vi "Facade.vi"(0 "Data In":T6, 2 "Display State In":T2, 3 "Container State":T5) -> (6 "Data Out":T6, 7 "Display State Out":T2, 8 "Action":T1)   [LabVIEW 2017, in "UI_TimeSelector.xctl"]
uses:
  UI_TimeSelector.xctl
  Data.ctl
  <vilib>/_xctls/Container State.ctl
  State.ctl
  Typedefs/INTERNAL-DATA.ctl
  Interface/DEF-Mode.ctl
  <vilib>/_xctls/Action.ctl
  Typedefs/INTERNAL-REFs.ctl
  <vilib>/_xctls/XControlSupport.lvlib
panel:
  in  "Second":string(combo)
  in  "Year":string(combo)
  in  "Month":string(combo)
  in  "Day":string(combo)
  in  "Hour":string(combo)
  in  "Minute":string(combo)
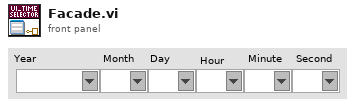
[diagram p1: front panel]
types:
  T1 = typedef "XControlSupport.lvlib/Action.ctl" = cluster{"Data Changed?":bool, "State Changed?":bool, "Action Name":string}
  T2 = typedef "UI_TimeSelector.xctl/State.ctl" = cluster{"data":T3, "mode":T4}
  T3 = typedef "UI_TimeSelector.xctl/INTERNAL-DATA.ctl" = cluster{"year":string, "month":string, "day":string, "hour":string, "minute":string, "second":string}
  T4 = typedef "UI_TimeSelector.xctl/DEF-Mode.ctl" = enum16{"YYYYMMDDHHMM", "YYYYMMDDHHMMSS", "YYYY", "YYYYMM", "YYYYMMDD", "HHMM", "HHMMSS"}
  T5 = typedef "XControlSupport.lvlib/Container State.ctl" = cluster{"Indicator?":bool, "Run Mode?":bool, " Refnum":refnum<vi>}
  T6 = typedef "UI_TimeSelector.xctl/Data.ctl" = timestamp
  T7 = typedef "UI_TimeSelector.xctl/INTERNAL-REFs.ctl" = cluster{"Year":refnum<vi>, "Month":refnum<vi>, "Day":refnum<vi>, "Hour":refnum<vi>, "Minute":refnum<vi>, "Second":refnum<vi>}
  T8 = cluster{"Year":string, "Month":string, "Day":string, "Hour":string, "Minute":string, "Second":string}
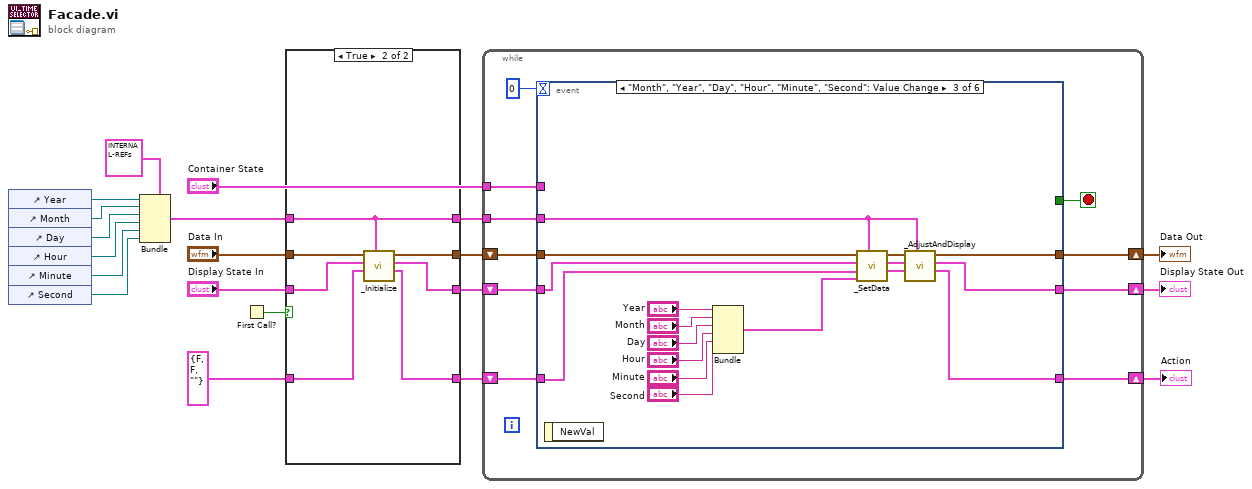
[diagram p0: block diagram]
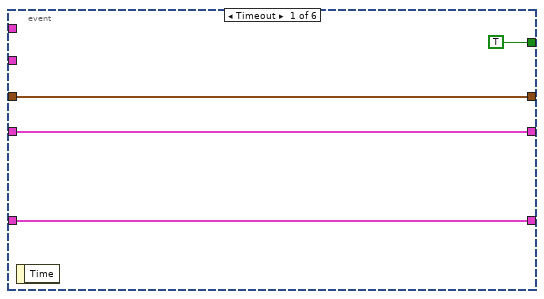
[diagram p3: hidden frame]
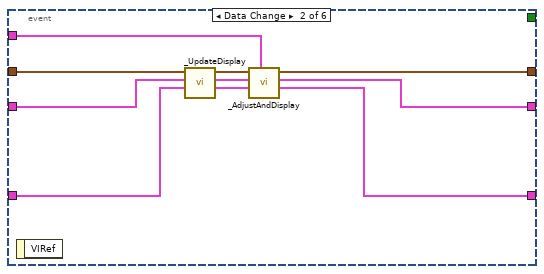
[diagram p4: hidden frame]
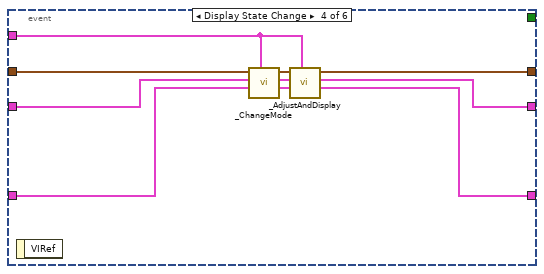
[diagram p5: hidden frame]
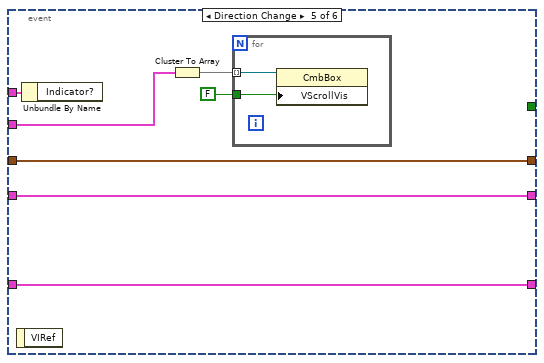
[diagram p6: hidden frame]
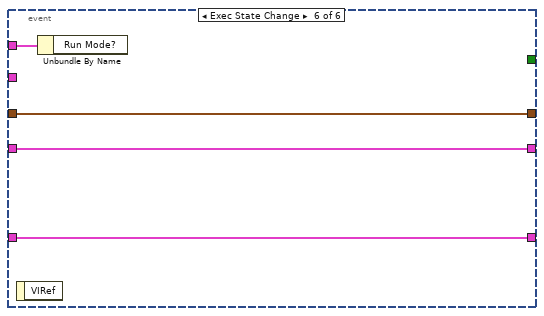
[diagram p7: hidden frame]
diagram:
  n1 = control-ref of="Year"() -> (w12:refnum<vi>)
  n2 = control-ref of="Month"() -> (w11:refnum<vi>)
  n3 = control-ref of="Day"() -> (w10:refnum<vi>)
  n4 = control-ref of="Hour"() -> (w9:refnum<vi>)
  n5 = control-ref of="Minute"() -> (w8:refnum<vi>)
  n6 = control-ref of="Second"() -> (w7:refnum<vi>)
  n7 = Bundle(cluster=T7 {"Year"=refnum, "Month"=refnum, "Day"=refnum, "Hour"=refnum, "Minute"=refnum, "Second"=refnum}, "Year"=w12, "Month"=w11, "Day"=w10, "Hour"=w9, "Minute"=w8, "Second"=w7) -> (w13:T7)
  n8 = First Call?() -> (First Call?: T/F=w2:bool)
  n9 = case shown="True" w2 {
    tunnel: [w23 w31] -> w19
    tunnel: [w24 w30] -> w16
    tunnel: [w21 w29] -> w14
    tunnel: w13 -> [w22 w25]
    tunnel: T1 {"Data Changed?"=FALSE, "State Changed?"=FALSE, "Action Name"=""} ("Action") -> [w21 w28]
    tunnel: "Data In" -> [w23 w27]
    tunnel: "Display State In" -> [w24 w26]
    tunnel: [w22 w25] -> w1
    frame False {
    }
    frame True {
      n10 = call "_Initialize.vi"("Refs"=w25, "Action in"=w28, "Display State In in"=w26, "Data In in"=w27) -> ("Action out"=w29:T1, "Display State In out"=w30:T2, "Data In out"=w31:T6)  [unwired: 5 in]
    }
  }
  n11 = while {
    shift-right: [w40] -> w17
    shift-left: w16 -> [w41]
    tunnel: "Container State" -> [w37]
    shift-right: [w32] -> w20
    shift-left: w19 -> [w36]
    shift-right: [w34] -> w15
    shift-left: w14 -> [w35]
    tunnel: w1 -> [w33]
    stop <- w39 stop-if-true
    n12 = event shown="[2] \"Month\", \"Year\", \"Day\", \"Hour\", \"Minute\", \"Second\": Value Change" {
      selector: _ -> [_ _ _ _ _ _]
      dyn-events: _ -> [_ _ _ _ _ _]
      timeout: 0 -> [_ _ _ _ _ _]
      tunnel: w41 -> [w42 w55 w56 w81 w88 w94]
      tunnel: [w42 w49 w70 w74 w88 w94] -> w40
      tunnel: [TRUE _ _ _ _ _] -> w39
      tunnel: w37 -> [_ _ _ _ w89 w95]
      tunnel: w36 -> [w44 w53 w59 w82 w83 w92]
      tunnel: [w43 w46 w71 w73 w87 w93] -> w34
      tunnel: w35 -> [w43 w54 w58 w80 w87 w93]
      tunnel: w33 -> [_ w51 w62 w77 w86 _]
      tunnel: [w44 w50 w72 w78 w83 w92] -> w32
      event Timeout {
        n13 = event-data() -> ()  [unwired: 1 in, 1 out]
      }
      event Data Change {
        n14 = event-data() -> ()  [unwired: 1 in, 1 out]
        n15 = call "_UpdateDisplay.vi"("Action in"=w54, "Display State In in"=w55, "Data In in"=w53) -> ("Action out"=w47:T1, "Display State In out"=w48:T2, "Data In out"=w52:T6)  [unwired: 6 in]
        n16 = call "_AdjustAndDisplay.vi"("Refs"=w51, "Action in"=w47, "Display State In in"=w48, "Data In in"=w52) -> ("Action out"=w46:T1, "Display State In out"=w49:T2, "Data In out"=w50:T6)  [unwired: 5 in]
      }
      event "Month", "Year", "Day", "Hour", "Minute", "Second": Value Change {
        n17 = event-data() -> ()  [unwired: 1 in, 1 out]
        n18 = Bundle("Year"="Year", "Month"="Month", "Day"="Day", "Hour"="Hour", "Minute"="Minute", "Second"="Second") -> (w57:T8)  [unwired: 1 in]
        n19 = call "_SetData.vi"("Refs"=w62, "data"=w57, "Action in"=w58, "Display State In in"=w56, "Data In in"=w59) -> ("Action out"=w60:T1, "Display State In out"=w61:T2, "Data In out"=w63:T6)  [unwired: 4 in]
        n20 = call "_AdjustAndDisplay.vi"("Refs"=w62, "Action in"=w60, "Display State In in"=w61, "Data In in"=w63) -> ("Action out"=w71:T1, "Display State In out"=w70:T2, "Data In out"=w72:T6)  [unwired: 5 in]
      }
      event Display State Change {
        n21 = event-data() -> ()  [unwired: 1 in, 1 out]
        n22 = call "_ChangeMode.vi"("refs"=w77, "Action in"=w80, "Display State In in"=w81, "Data In in"=w82) -> ("Action out"=w75:T1, "Display State In out"=w76:T2, "Data In out"=w79:T6)  [unwired: 4 in, 1 out]
        n23 = call "_AdjustAndDisplay.vi"("Refs"=w77, "Action in"=w75, "Display State In in"=w76, "Data In in"=w79) -> ("Action out"=w73:T1, "Display State In out"=w74:T2, "Data In out"=w78:T6)  [unwired: 5 in]
      }
      event Direction Change {
        n24 = event-data() -> ()  [unwired: 1 in, 1 out]
        n25 = Unbundle By Name(w89) -> ()  [unwired: 1 out]
        n26 = Cluster To Array(cluster=w86) -> (array=w85:refnum<vi>[])
        n27 = for {
          tunnel: w85 -> [w91] mode=indexing
          tunnel: FALSE -> [w90]
          n28 = property class="CmbBox"(reference=w91, "VScrollVis"=w90) -> ()  [unwired: 1 in, 2 out]
        }
      }
      event Exec State Change {
        n29 = event-data() -> ()  [unwired: 1 in, 1 out]
        n30 = Unbundle By Name(w95) -> ()  [unwired: 1 out]
      }
    }
  }
  "Display State Out" <- w17
  "Data Out" <- w20
  "Action" <- w15
